vi "Close Hardware.vi"(8 "error in (no error)":errorcluster, 11 "Instrument.Aerotech in":refnum<class "Instrument.Aerotech.lvclass">) -> (0 "error out":errorcluster, 3 "Instrument.Aerotech out":refnum<class "Instrument.Aerotech.lvclass">)   [LabVIEW 2019, in "Instrument.Aerotech.lvclass"]
uses:
  Instrument.Aerotech.lvclass
  Instrument.Aerotech.lvclass/Instrument.Aerotech.ctl
  C:/Users/patrick/Documents/GitHub/levylabpitt/Aerotech-Delay-Line/lvsrc/Aerotech-Ensemble-LabVIEW/2010-5.6/Bin/Aerotech.Ensemble.dll
  Aerotech-Ensemble-LabVIEW/2010-5.6/Bin/Aerotech.Ensemble.dll
  Aerotech-Ensemble-LabVIEW/2010-5.6/Motion/AbortSingle.vi
  Aerotech-Ensemble-LabVIEW/2010-5.6/Motion/DisableSingle.vi
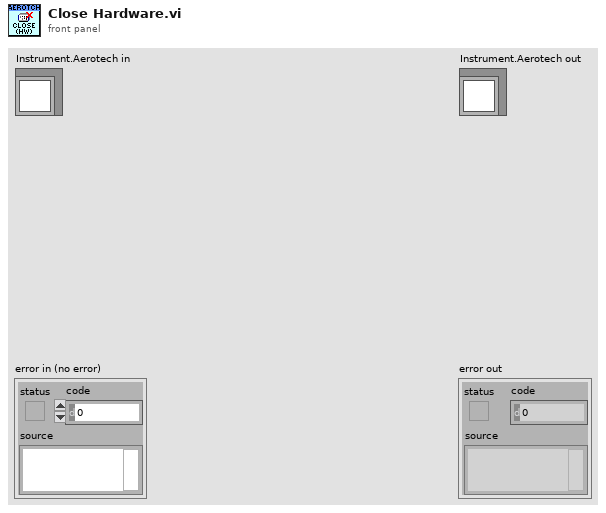
[diagram p1: front panel]
types:
  T1 = typedef "ControllerDiagPacket.ctl" = cluster{"Count":i32, "Packet Time":i64, "Axes":T2[], "error":errorcluster}
  T2 = typedef "AxisDiagPacket.ctl" = cluster{"Axis Name":string, "Acceleration Command":dbl, "Amplifier Temperature":sgl, "Analog Input 0":dbl, "Analog Input 1":dbl, "Analog Output 0":dbl, "Analog Output 1":dbl, "Axis Fault (num)":i32, "Axis Fault (str)":string, "Axis Fault (bits)":cluster{"AmplifierFault":bool, "AmplifierTemperatureFault":bool, "CcwEndOfTravelLimitFault":bool, "CcwSoftwareLimitFault":bool, "CommunicationLostFault":bool, "CwEndOfTravelLimitFault":bool, "CwSoftwareLimitFault":bool, "EmergencyStopFault":bool, "EncoderFault":bool, "ExternalFault":bool, "FeedbackScalingFault":bool, "HallSensorFault":bool, "MarkerSearchFault":bool, "MaxVelocityCommandFault":bool, "MotorTemperatureFault":bool, "None":bool, "OverCurrentFault":bool, "PositionErrorFault":bool, "PositionFeedbackFault":bool, "PowerSupplyFault":bool, "VelocityErrorFault":bool, "VelocityFeedbackFault":bool, "VoltageClampFault":bool}, "Axis Status (num)":i32, "Axis Status (str)":string, "Axis Status (bits)":cluster{"AccelerationPhase":bool, "AutofocusActive":bool, "BrakeOutput":bool, "CalibrationActive":bool, "CalibrationEnabled":bool, "CcwEndOfTravelLimitInput":bool, "CommandShapingFilterDone":bool, "CosineEncoderError":bool, "CurrentClamp":bool, "CwEndOfTravelLimitInput":bool, "DecelerationPhase":bool, "EmergencyStopInput":bool, "Enabled":bool, "GantryMasterActive":bool, "GantryModeActive":bool, "HallAInput":bool, "HallBInput":bool, "HallCInput":bool, "Homed":bool, "HomeLimitInput":bool, "Homing":bool, "InPosition":bool, "InPosition2":bool, "JoystickControl":bool, "MarkerInput":bool, "MasterMotionSuppressed":bool, "MasterSlaveControl":bool, "MotionIsCw":bool, "MoveActive":bool, "None":bool, "PositionCaptureActive":bool, "ServoControl":bool, "SineEncoderError":bool}, "Current Command":sgl, "Current Error":sgl, "Current Feedback":sgl, "Digital Input 0":i32, "Digital Input 1":i32, "Digital Input 2":i32, "Digital Output 0":i32, "Digital Output 1":i32, "Digital Output 2":i32, "Position Feedback Auxiliary":dbl, "Position Command":dbl, "Position Error":dbl, "Position Feedback":dbl, "Program Position Command":dbl, "Program Position Error":dbl, "Program Position Feedback":dbl, "Velocity Command":dbl, "Velocity Error":dbl, "Velocity Feedback":dbl}
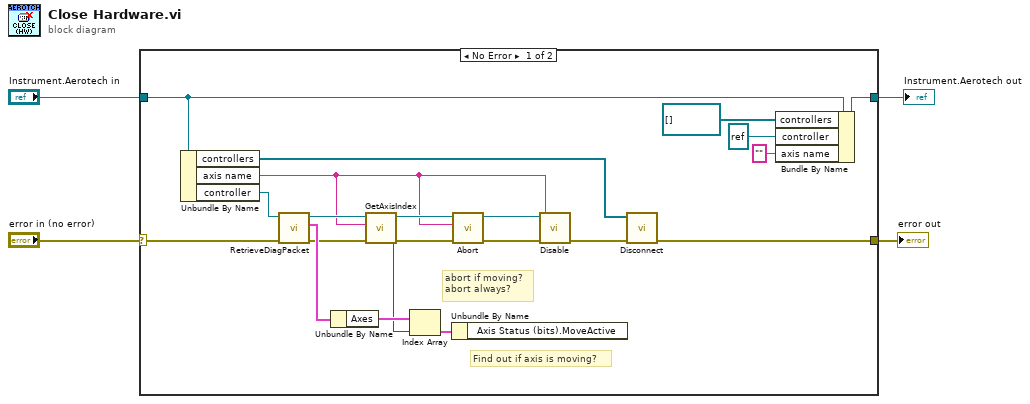
[diagram p0: block diagram]
diagram:
  n1 = case shown="No Error" "error in (no error)" {
    selector: "error in (no error)" -> [w6 w26]
    tunnel: [w13 w26] -> w4
    tunnel: "Instrument.Aerotech in" -> [w12 w27]
    tunnel: [w11 w27] -> w2
    frame No Error {
      # "abort if moving?\nabort always?"
      # "Find out if axis is moving?"
      n2 = Unbundle By Name(w12) -> ("controllers"=w10:refnum<k24>[], "axis name"=w5:string, "controller"=w19:refnum<k24>)
      n3 = call "RetrieveDiagPacket.vi"("error in (no error)"=w6, "Controller In"=w19) -> ("error out"=w23:errorcluster, "ControllerDiagPacket"=w24:T1, "Controller Out"=w22:refnum<k24>)  [unwired: 7 in]
      n4 = Unbundle By Name(w24) -> ("Axes"=w21:T2[])
      n5 = call "GetAxisIndex.vi"("error in (no error)"=w23, "axis name"=w5, "controller in"=w22) -> ("error out"=w16:errorcluster, "axis index"=w18:i32, "controller out"=w17:refnum<k24>)  [unwired: 6 in]
      n6 = Index Array(array=w21, index=w18) -> (element=w20:T2)
      n7 = Unbundle By Name(w20) -> ()  [unwired: 1 out]
      n8 = call-poly "Abort.vi"("error in (no error)"=w16, "axis name? (all)"=w5, "controller in"=w17) -> ("error out"=w15:errorcluster, "controller out"=w14:refnum<k24>)  [unwired: 7 in]
      n9 = call-poly "Disable.vi"("error in (no error)"=w15, "axis name"=w5, "controller in"=w14) -> ("error out"=w25:errorcluster)  [unwired: 7 in, 1 out]
      n10 = call "Disconnect.vi"("error in (no error)"=w25, "controllers"=w10) -> ("error out"=w13:errorcluster)  [unwired: 9 in]
      n11 = Bundle By Name(cluster=w12, "controllers"=refnum<k24>[] [], "controller"=refnum<k24> refnum, "axis name"="") -> (w11:refnum<class "Instrument.Aerotech.lvclass">)
    }
    frame Error {
    }
  }
  "error out" <- w4
  "Instrument.Aerotech out" <- w2
